vi "Take Measurement.vi"(6 "Angle of Attack":dbl, 8 "Setup filename":string="Wing_Pressure.xls", 9 "Averaging time (min)":dbl, 10 "File":T1, 11 "Filename":path) -> (0 "Array":cluster{dbl[], dbl[]}[](array[cluster]), 1 "Uref":dbl format="%#.3f", 2 "U Trav":dbl, 3 "Z":dbl)   [LabVIEW 2022 SP3]
uses:
  Anemometry/Anemometry Sub Vis/Controls/Save_Data.ctl
  Camera Server/Camera enum/Camera resolution.ctl
  Anemometry/Anemometry Sub Vis/Controls/Setup.ctl
  Anemometry/Anemometry Sub Vis/Globals/Meas_global.vi
  <vilib>/gmath/NI_Gmath.lvlib
panel:
  out "Lift/Drag":dbl format="%#.3f"
  out "CD":dbl format="%.3f"
  out "CL":dbl format="%.3f"
  out "Drag (N)":dbl format="%.3f"
  out "Lift (N)":dbl format="%.3f"
  out "Density Kg/m^3":dbl format="%#.3f"
  out "Fx Lower":dbl format="%#.3f"
  out "Fx Upper":dbl format="%#.3f"
  out "Fy Lower":dbl format="%#.2f"
  out "Fy Upper":dbl format="%#.2f"
  out "Fx (N)":dbl format="%.3f"
  out "Fy (N)":dbl format="%.3f"
  out "Fx":cluster{"xi used":dbl[], dbl[]}[](graph)
  out "Fy":cluster{"xi used":dbl[], dbl[]}[](graph)
  out "Pressure":cluster{dbl[], dbl[]}[](graph)
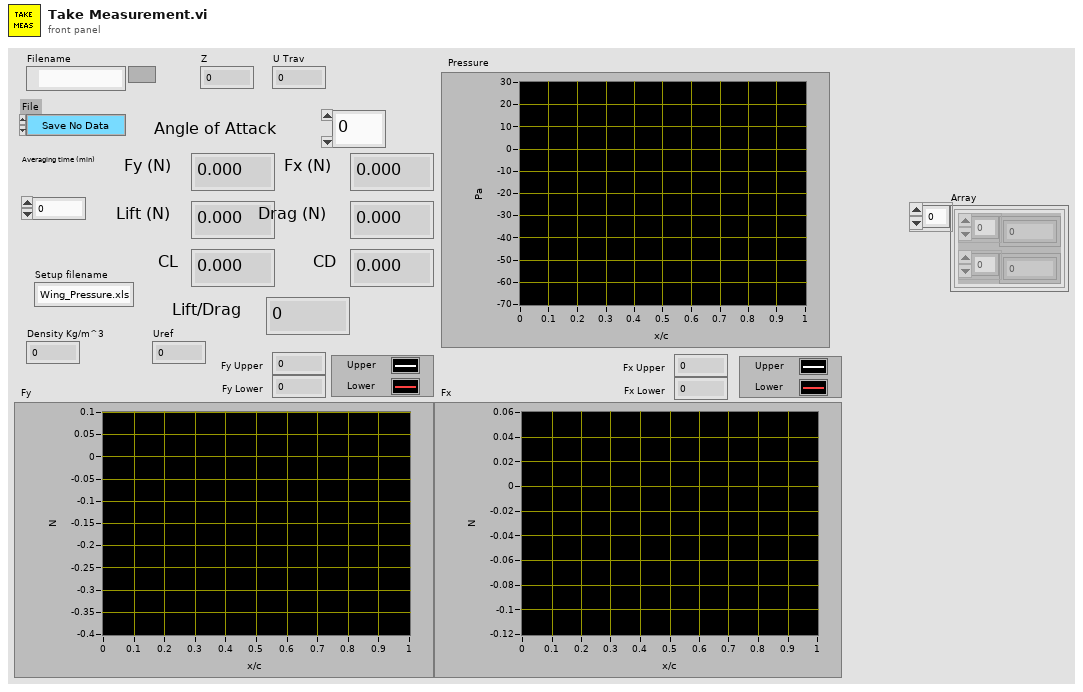
[diagram p1: front panel]
types:
  T1 = typedef "Save_Data.ctl" = enum16{"Save No Data", "Save Data"}
  T2 = typedef "Setup.ctl" = enum16{"Run Program", "Show Setup", "Save Current Setup", "Setup Front Panel"}
  T3 = typedef "Camera resolution.ctl" = u8
  T4 = typedef "Analysis_info_cluster.ctl" = cluster{"Colour":u32, "Inst type":T5, "Inst name":string, "Symbol":string, "Code name":string, "Extra Info":string, "Inst Array":T6, "Extra Titles":string[], "Extra Values":string[], "U":dbl, "u^2":dbl, "u^3":dbl, "u^4":dbl, "Skew_u":dbl, "Kurt_u":dbl, "Sd Error in Mean":dbl, "% u'/U":dbl, "X":dbl, "Y":dbl, "Z":dbl, "Timescale integral Estimate":dbl, "Sd Error in Variance":dbl, "Calib File":path, "Calib Constants":dbl[], "Output Position":bool, "Stats":enum16{"None", "Basic", "Full"}, "Av Sampling Rate":dbl, "Av No of Samples":dbl, "Total Meas Time (s)":dbl, "ADAM Ch Name":string, "Max value":dbl, "Min value":dbl, "Req Sample Rate Hz":dbl, "Sync Delay Time (s)":dbl, "Ch No":i16, "Device":string, "Use Latest Calib":bool, "Port":string, "Metadata Ch Names":string[], "Metadata Ch Values":string[], "Label":string}
  T5 = typedef "Inst_type.ctl" = enum16{"Raw voltage", "Raw with zero offsetting", "Propeller anemometer", "Pressure Transducer", "Pitot-static tube", "Hot wire", "Cross wire 1", "Cross wire 2", "Generic Linear", "Generic Polynomial", "Generic BackPoly", "Fast FID", "Thermocouple", "Cold wire", "Pulsed Wire", "LDA Vel", "LDA Tran time", "LDA Arr time", "Microphone"}
  T6 = typedef "Instrument_Array.ctl" = enum16{"PWA", "LDA", "Analogue"}
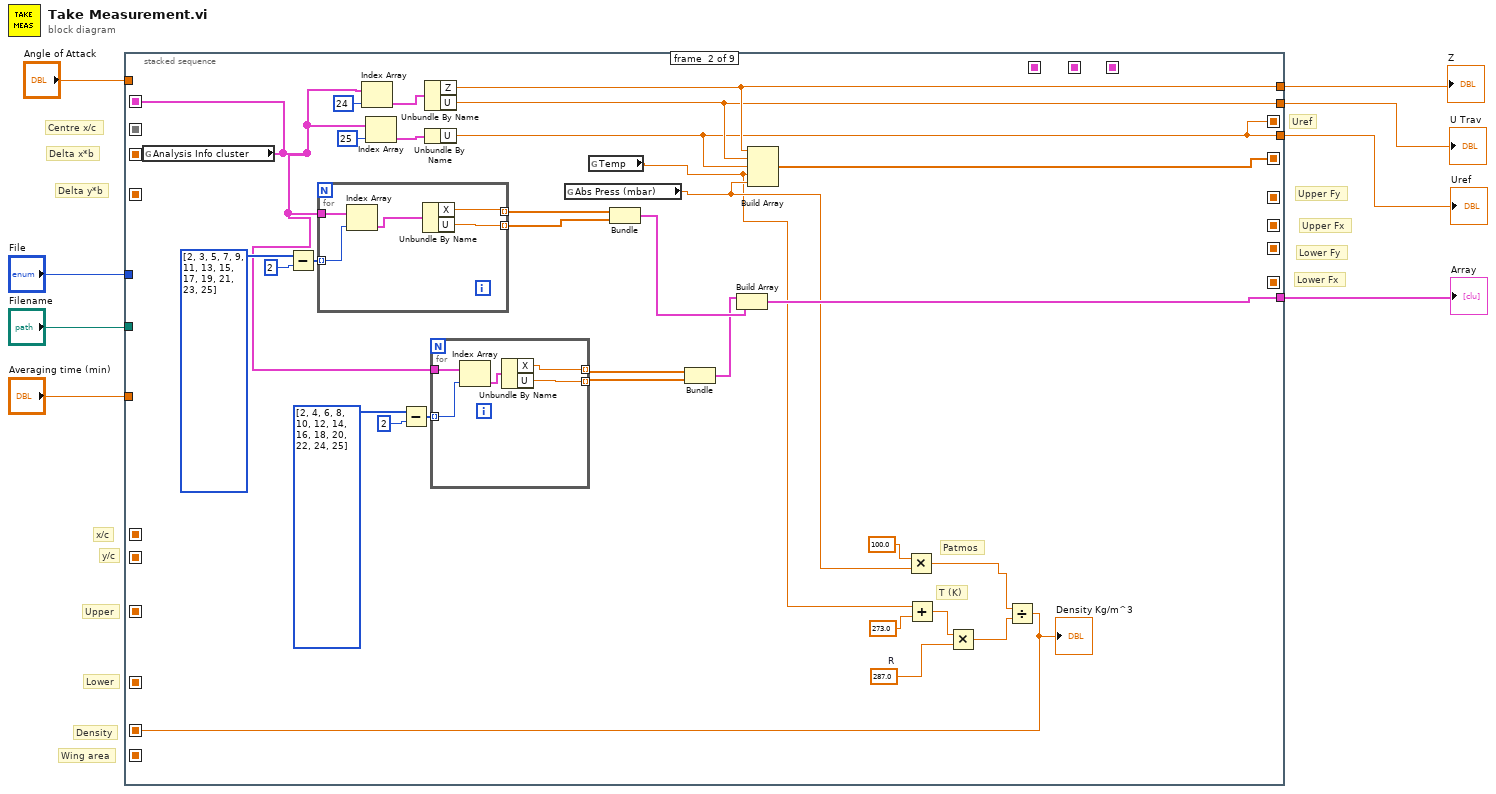
[diagram p0: block diagram]
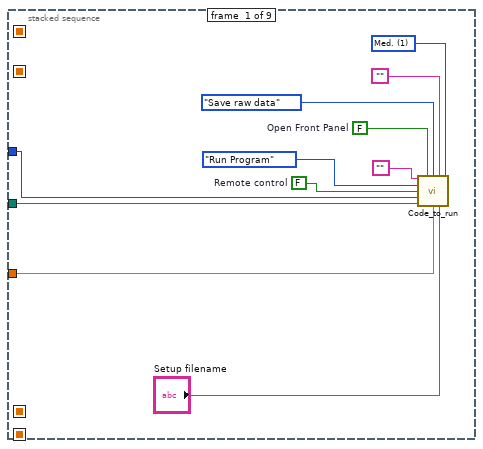
[diagram p2: hidden frame]
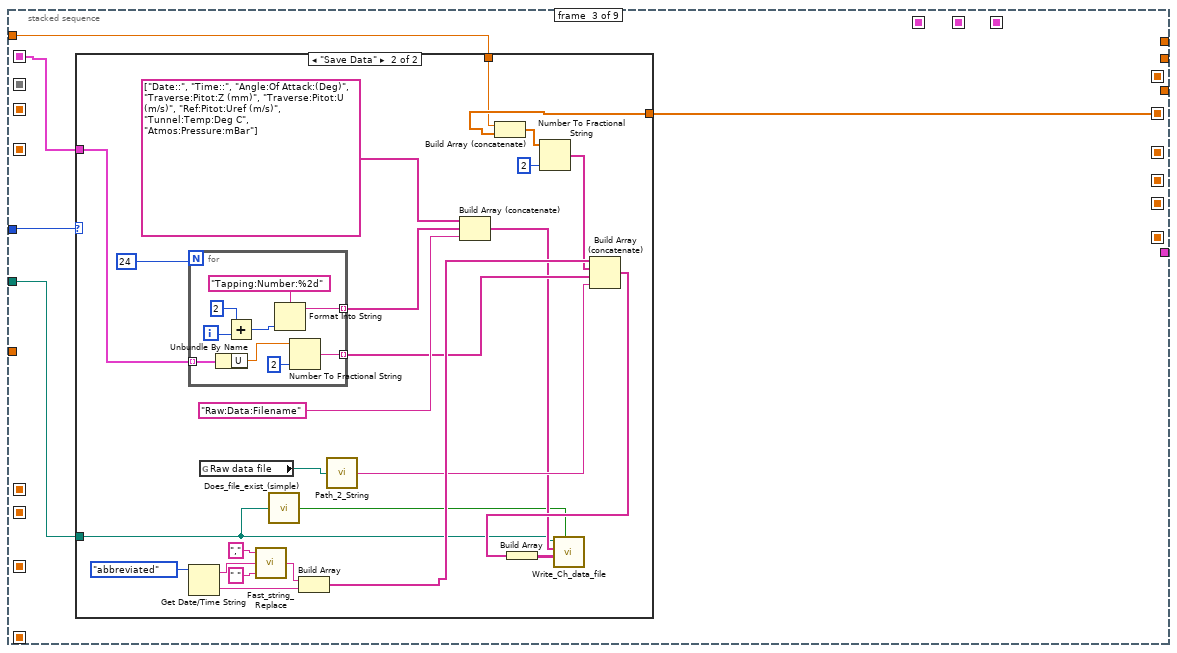
[diagram p3: hidden frame]
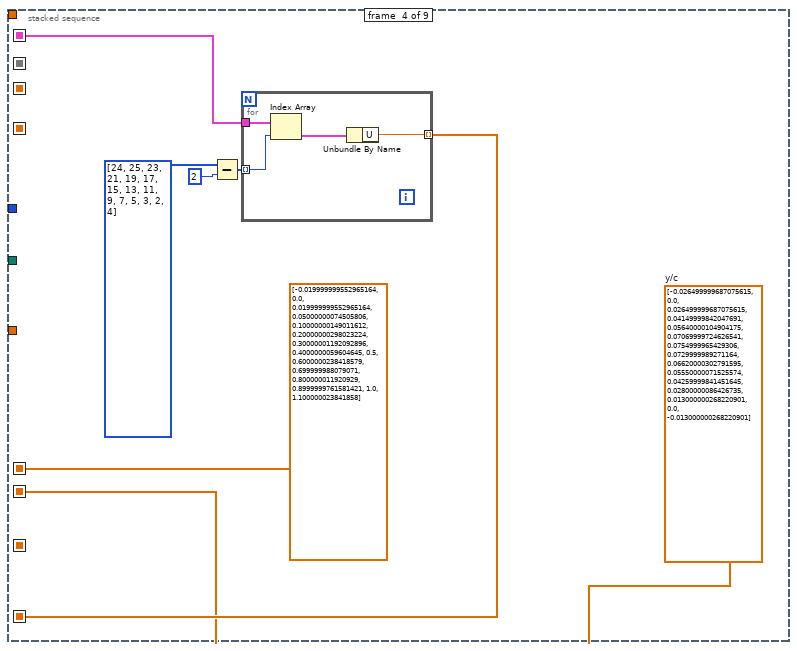
[diagram p5: hidden frame]
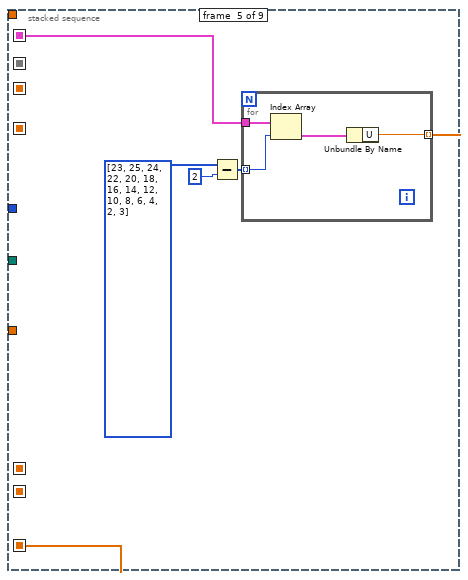
[diagram p6: hidden frame]
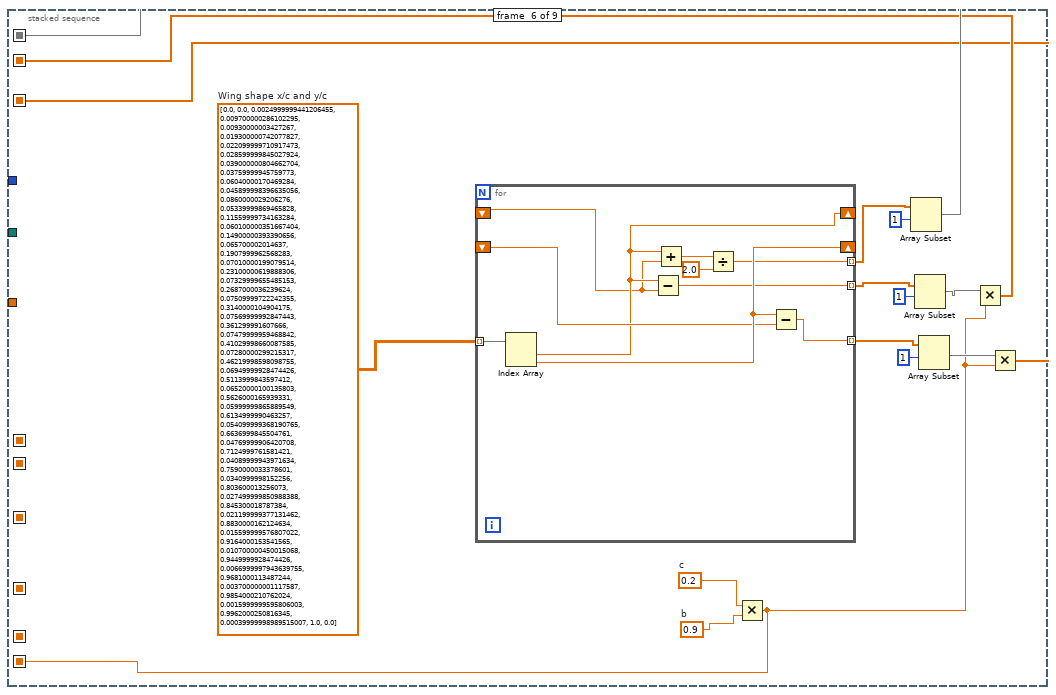
[diagram p7: hidden frame]
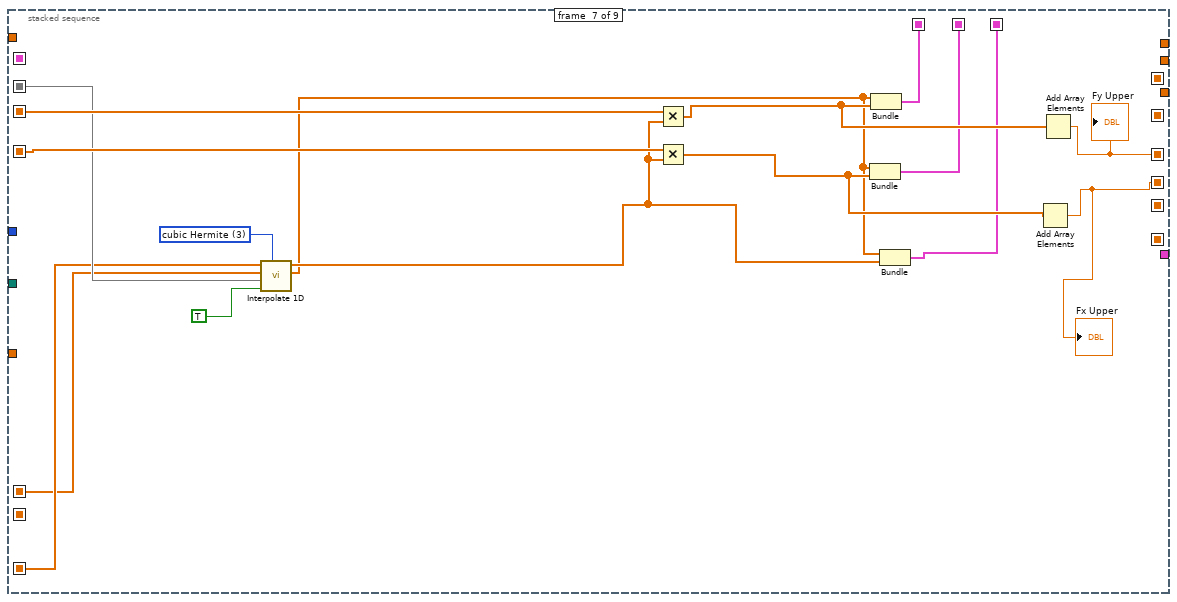
[diagram p8: hidden frame]
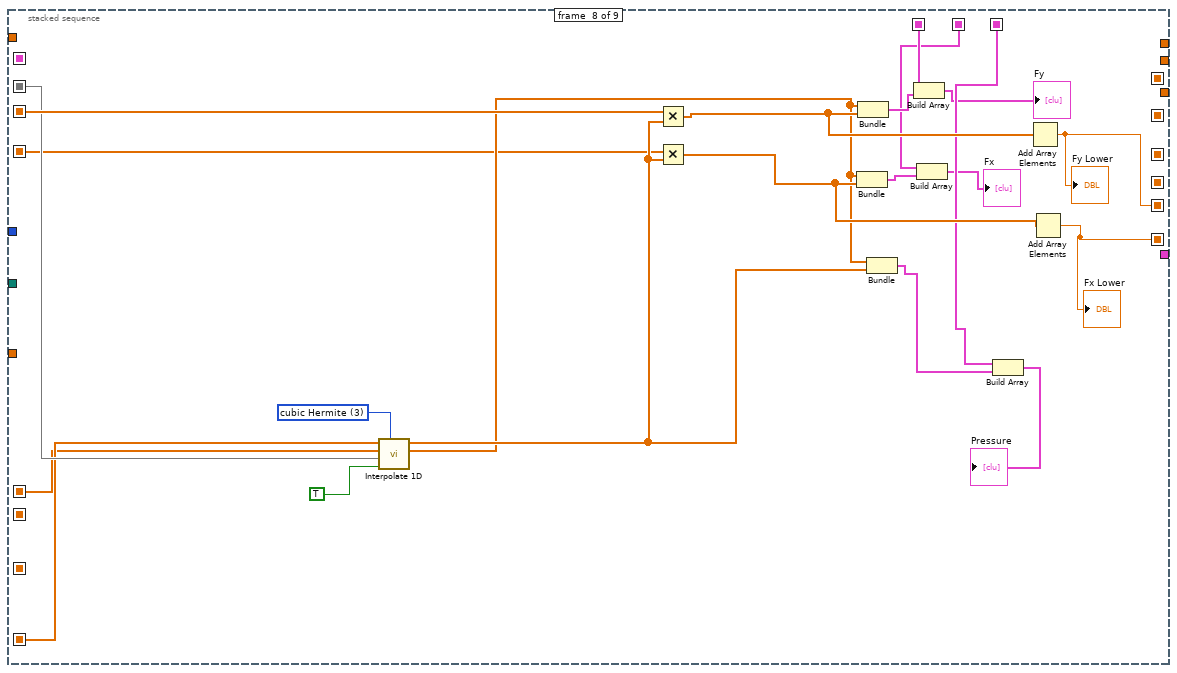
[diagram p9: hidden frame]
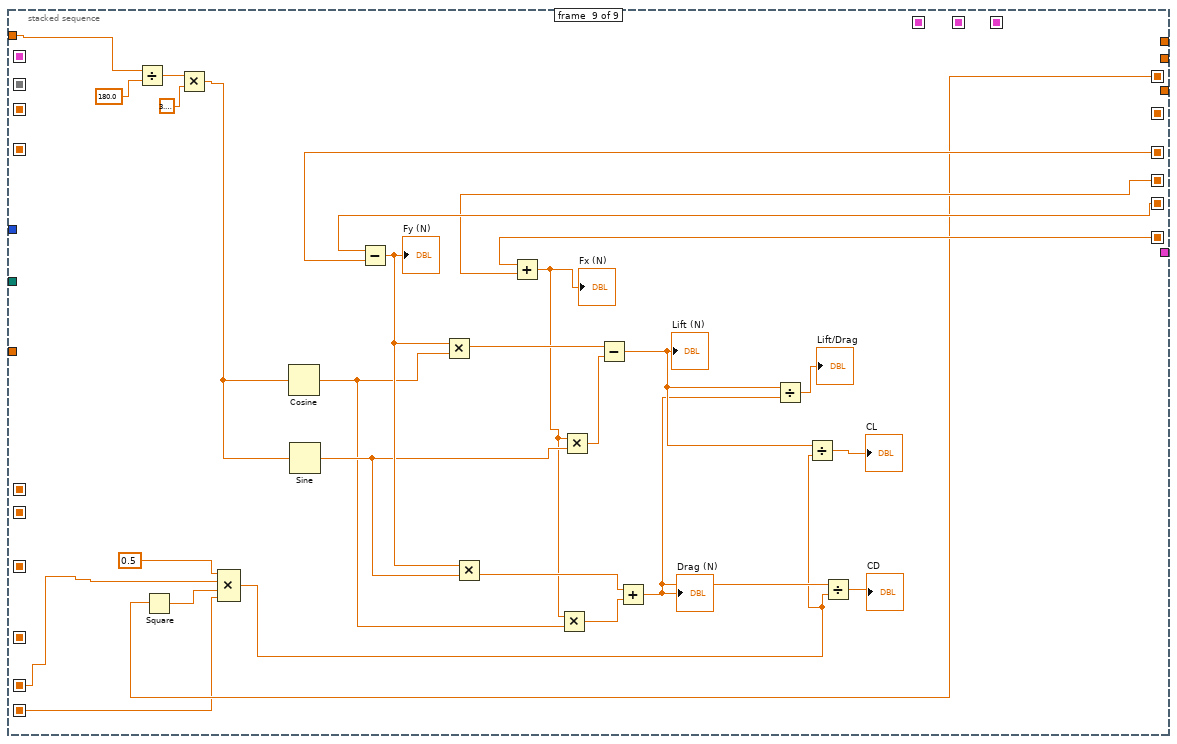
[diagram p10: hidden frame]
diagram:
  # "Wing area"
  # "Uref"
  # "Density"
  # "Lower Fx"
  # "Lower Fy"
  # "Upper Fx"
  # "Upper Fy"
  # "Delta y*b"
  # "Delta x*b"
  # "Centre x/c"
  # "y/c"
  # "x/c"
  # "Upper"
  # "Lower"
  n1 = stacked-sequence {
    seq-local: [_ w38 _ _ _ _ _ _ _] -> [_ _ w64 w103 w112 _ _ _ _]
    seq-local: [_ w32 _ _ _ _ _ _ _] -> [_ _ w63 _ _ _ _ _ _]
    seq-local: [_ _ _ w102 _ _ _ _ _] -> [_ _ _ _ _ _ _ w176 _]
    seq-local: [_ _ _ _ w111 _ _ _ _] -> [_ _ _ _ _ _ w152 _ _]
    seq-local: [_ _ _ dbl[] [-0.019999999552965164, 0.0, 0.019999999552965164, 0.05000000074505806, 0.10000000149011612, 0.20000000298023224, 0.30000001192092896, 0.4000000059604645, 0.5, 0.6000000238418579, 0.699999988079071, 0.800000011920929, 0.8999999761581421, 1.0, 1.100000023841858] _ _ _ _ _] -> [_ _ _ _ _ _ w151 w175 _]
    seq-local: [_ _ _ w100 _ _ _ _ _] -> [_ _ _ _ _ _ _ _ _]
    seq-local: [_ _ _ _ _ w131 _ _ _] -> [_ _ _ _ _ _ w158 w181 _]
    seq-local: [_ _ _ _ _ w123 _ _ _] -> [_ _ _ _ _ _ w160 w182 _]
    seq-local: [_ _ _ _ _ w121 _ _ _] -> [_ _ _ _ _ _ w159 w161 _]
    seq-local: [_ _ _ _ _ _ w156 _ _] -> [_ _ _ _ _ _ _ _ w209]
    seq-local: [_ _ _ _ _ _ w145 _ _] -> [_ _ _ _ _ _ _ _ w208]
    seq-local: [_ _ _ _ _ _ _ w163 _] -> [_ _ _ _ _ _ _ _ w210]
    seq-local: [_ _ _ _ _ _ _ w162 _] -> [_ _ _ _ _ _ _ _ w207]
    seq-local: [_ _ _ _ _ _ w148 _ _] -> [_ _ _ _ _ _ _ w167 _]
    seq-local: [_ _ _ _ _ _ w147 _ _] -> [_ _ _ _ _ _ _ w165 _]
    seq-local: [_ _ _ _ _ _ w146 _ _] -> [_ _ _ _ _ _ _ w170 _]
    seq-local: [_ w23 _ _ _ _ _ _ _] -> [_ _ _ _ _ _ _ _ w186]
    seq-local: [_ w22 _ _ _ _ _ _ _] -> [_ _ _ _ _ _ _ _ w185]
    seq-local: [_ _ _ _ _ w120 _ _ _] -> [_ _ _ _ _ _ _ _ w183]
    tunnel: "Filename" -> [w12 _ w62 _ _ _ _ _ _]
    tunnel: [_ w41 _ _ _ _ _ _ _] -> w3
    tunnel: [_ w22 _ _ _ _ _ _ _] -> w4
    tunnel: [_ w33 _ _ _ _ _ _ _] -> w5
    tunnel: [_ w34 _ _ _ _ _ _ _] -> w6
    tunnel: "Averaging time (min)" -> [w11 _ _ _ _ _ _ _ _]
    tunnel: "File" -> [w10 _ w65 _ _ _ _ _ _]
    tunnel: "Angle of Attack" -> [_ _ w61 _ _ _ _ _ w206]
    frame #0 {
      w17 = FALSE  # Remote control
      w14 = FALSE  # Open Front Panel
      w19 = T3 1 items=["Low", "Med.", "High", "Max."] ("Camera Resolution")
      n2 = call "Code_to_run.vi"("Extra command String"="", "Open Front Panel"=w14, "Raw data option"=enum16{"Save raw data", "Raw data not saved"}."Save raw data", "Current Row Comments"="", "Camera Resolution"=w19, "setup"=Setup."Run Program", "Remote control"=w17, "File"=w10, "Results Filename"=w12, "Averaging time (min)"=w11, "Setup filename"="Setup filename") -> ()  [unwired: 4 in, 1 out]
    }
    frame #1 {
      w26 = 287.0  # R
      # "T (K)"
      # "Patmos"
      n3 = global read "Meas_global.vi" "Analysis Info cluster"() -> (w38:T4[])
      n4 = Subtract(x=i32[] [2, 3, 5, 7, 9, 11, 13, 15, 17, 19, 21, 23, 25], y=2) -> (x-y=w49:i32[])
      n5 = for {
        tunnel: w38 -> [w60]
        tunnel: w49 -> [w59] mode=indexing
        tunnel: [w57] -> w37 mode=indexing
        tunnel: [w56] -> w46 mode=indexing
        n6 = Index Array(array=w60, index=w59) -> (element=w58:T4)
        n7 = Unbundle By Name(w58) -> ("X"=w56:dbl, "U"=w57:dbl)
      }
      n8 = Index Array(array=w38, index=24) -> (element=w42:T4)
      n9 = Index Array(array=w38, index=25) -> (element=w44:T4)
      n10 = Subtract(x=i32[] [2, 4, 6, 8, 10, 12, 14, 16, 18, 20, 22, 24, 25], y=2) -> (x-y=w48:i32[])
      n11 = Unbundle By Name(w42) -> ("Z"=w34:dbl, "U"=w33:dbl)
      n12 = Unbundle By Name(w44) -> ("U"=w22:dbl)
      n13 = for {
        tunnel: w38 -> [w55]
        tunnel: w48 -> [w54] mode=indexing
        tunnel: [w52] -> w35 mode=indexing
        tunnel: [w51] -> w36 mode=indexing
        n14 = Index Array(array=w55, index=w54) -> (element=w53:T4)
        n15 = Unbundle By Name(w53) -> ("X"=w51:dbl, "U"=w52:dbl)
      }
      n16 = global read "Meas_global.vi" "Abs Press (mbar)"() -> (w31:dbl)
      n17 = global read "Meas_global.vi" "Temp"() -> (w29:dbl)
      n18 = Bundle(w46, w37) -> (w21:cluster{dbl[], dbl[]})  [unwired: 1 in]
      n19 = Bundle(w36, w35) -> (w20:cluster{dbl[], dbl[]})  [unwired: 1 in]
      n20 = Build Array(w20, w21) -> (w41:cluster{dbl[], dbl[]}[])
      n21 = Build Array(w34, w33, w22, w29, w31) -> (w32:dbl[])
      n22 = Multiply(x=100.0, y=w31) -> (x*y=w24:dbl)
      n23 = Add(x=w29, y=273.0) -> (x+y=w27:dbl)
      n24 = Multiply(x=w27, y=w26) -> (x*y=w25:dbl)
      n25 = Divide(x=w24, y=w25) -> (x/y=w23:dbl)
      "Density Kg/m^3" <- w23
    }
    frame #2 {
      n26 = case shown="\"Save Data\"" w65 {
        tunnel: w64 -> [_ w77]
        tunnel: w63 -> [_ w70]
        tunnel: w62 -> [_ w68]
        tunnel: w61 -> [_ w66]
        frame "Save No Data", Default {
        }
        frame "Save Data" {
          n27 = for {
            N: 24 -> [_]
            tunnel: [w95] -> w88 mode=indexing
            tunnel: w77 -> [w94] mode=indexing
            tunnel: [w91] -> w76 mode=indexing
            i -> [w99]
            n28 = Unbundle By Name(w94) -> ("U"=w92:dbl)
            n29 = Add(x=2, y=w99) -> (x+y=w97:i32)
            n30 = Format Into String(format string="Tapping:Number:%2d", w97) -> (resulting string=w95:string)  [unwired: 2 in, 1 out]
            n31 = Number To Fractional String(number=w92, precision (6)=i16 2) -> (F-format string=w91:string)  [unwired: 2 in]
          }
          n32 = Get Date/Time String(date format (0)=enum16{"short", "long", "abbreviated"}."abbreviated") -> (date string=w86:string, time string=w81:string)  [unwired: 2 out]
          n33 = global read "Meas_global.vi" "Raw data file"() -> (w75:path)
          n34 = call "Fast_string_Replace.vi"("Replace match with:"=" ", "Input String"=w86, "matchThis"="," ("regular expression")) -> ("Output String"=w82:string)  [unwired: 1 in, 1 out]
          n35 = call "Does_file_exist_(simple).vi"("Pathname"=w68) -> ("exists?"=w67:bool)
          n36 = Build Array(w82, w81) -> (w79:string[])
          n37 = call "Path_2_String.vi"("Real Path"=w75) -> ("Path String"=w74:string)
          n38 = Build Array (concatenate)(string[] ["Date::", "Time::", "Angle:Of Attack:(Deg)", "Traverse:Pitot:Z (mm)", "Traverse:Pitot:U (m/s)", "Ref:Pitot:Uref (m/s)", "Tunnel:Temp:Deg C", "Atmos:Pressure:mBar"], w88, "Raw:Data:Filename") -> (w71:string[])
          n39 = Build Array (concatenate)(w66, w70) -> (w69:dbl[])
          n40 = Number To Fractional String(number=w69, precision (6)=i16 2) -> (F-format string=w78:string[])  [unwired: 2 in]
          n41 = Build Array (concatenate)(w79, w78, w76, w74) -> (w73:string[])
          n42 = Build Array(w73) -> (w72:string[][])
          n43 = call "Write_Ch_data_file.vi"("exists?"=w67, "Channel Values"=w72, "Channel names"=w71, "Filename"=w68) -> ()  [unwired: 4 in, 4 out]
        }
      }
    }
    frame #3 {
      w100 = dbl[] [-0.026499999687075615, 0.0, 0.026499999687075615, 0.04149999842047691, 0.05640000104904175, 0.07069999724626541, 0.0754999965429306, 0.0729999989271164, 0.06620000302791595, 0.05550000071525574, 0.04259999841451645, 0.02800000086426735, 0.013000000268220901, 0.0, -0.013000000268220901]  # y/c
      n44 = Subtract(x=i32[] [24, 25, 23, 21, 19, 17, 15, 13, 11, 9, 7, 5, 3, 2, 4], y=2) -> (x-y=w105:i32[])
      n45 = for {
        tunnel: w103 -> [w110]
        tunnel: w105 -> [w109] mode=indexing
        tunnel: [w107] -> w102 mode=indexing
        n46 = Index Array(array=w110, index=w109) -> (element=w108:T4)
        n47 = Unbundle By Name(w108) -> ("U"=w107:dbl)
      }
    }
    frame #4 {
      n48 = Subtract(x=i32[] [23, 25, 24, 22, 20, 18, 16, 14, 12, 10, 8, 6, 4, 2, 3], y=2) -> (x-y=w114:i32[])
      n49 = for {
        tunnel: w112 -> [w119]
        tunnel: w114 -> [w118] mode=indexing
        tunnel: [w116] -> w111 mode=indexing
        n50 = Index Array(array=w119, index=w118) -> (element=w117:T4)
        n51 = Unbundle By Name(w117) -> ("U"=w116:dbl)
      }
    }
    frame #5 {
      w125 = 0.9  # b
      w126 = 0.2  # c
      w134 = sgl[][] [[0.0, 0.0], [0.0025, 0.0097], [0.0093, 0.0193], [0.0221, 0.0286], [0.039, 0.0376], [0.0604, 0.0459], [0.086, 0.0534], [0.1156, 0.0601], [0.149, 0.0657], [0.1908, 0.0701], [0.231, 0.0733], [0.2687, 0.0751], [0.314, 0.0757], [0.3613, 0.0748], [0.4103, 0.0728], [0.4622, 0.0695], [0.5114, 0.0652], [0.5626, 0.06], [0.6135, 0.0541], [0.6637, 0.0477], [0.7125, 0.0409], [0.759, 0.0341], [0.8036, 0.0275], [0.8453, 0.0212], [0.883, 0.0156], [0.9164, 0.0107], [0.945, 0.0067], [0.9681, 0.0037], [0.9854, 0.0016], [0.9962, 0.0004], [1.0, 0.0]]  # Wing shape x/c and y/c
      n52 = for {
        tunnel: w134 -> [w144] mode=indexing
        shift-right: [w141] -> _
        shift-left: _ -> [w140]
        shift-right: [w143] -> _
        shift-left: _ -> [w142]
        tunnel: [w137] -> w132 mode=indexing
        tunnel: [w136] -> w129 mode=indexing
        tunnel: [w135] -> w128 mode=indexing
        n53 = Index Array(array=w144) -> (element #1=w141:sgl, element #2=w143:sgl)  [unwired: 2 in]
        n54 = Subtract(x=w141, y=w140) -> (x-y=w136:sgl)
        n55 = Add(x=w141, y=w140) -> (x+y=w139:sgl)
        n56 = Divide(x=w139, y=sgl 2.0) -> (x/y=w137:sgl)
        n57 = Subtract(x=w143, y=w142) -> (x-y=w135:sgl)
      }
      n58 = Multiply(x=w126, y=w125) -> (x*y=w120:dbl)
      n59 = Array Subset(array=w132, index=1) -> (w131:sgl[])  [unwired: 1 in]
      n60 = Array Subset(array=w129, index=1) -> (w124:sgl[])  [unwired: 1 in]
      n61 = Array Subset(array=w128, index=1) -> (w122:sgl[])  [unwired: 1 in]
      n62 = Multiply(x=w124, y=w120) -> (x*y=w123:dbl[])
      n63 = Multiply(x=w122, y=w120) -> (x*y=w121:dbl[])
    }
    frame #6 {
      w154 = 3 items=["nearest", "linear", "spline", "cubic Hermite", "Lagrange"] ("method")
      n64 = call <vilib>:"Interpolate 1D.vi"("method"=w154, "X is monotonic"=TRUE, "xi"=w158, "X"=w151, "Y"=w152) -> ("xi used"=w149:dbl[], "yi"=w150:dbl[])  [unwired: 4 in, 1 out]
      n65 = Multiply(x=w160, y=w150) -> (x*y=w157:dbl[])
      n66 = Multiply(x=w159, y=w150) -> (x*y=w155:dbl[])
      n67 = Bundle("xi used"=w149, w155) -> (w147:cluster{"xi used":dbl[], dbl[]})  [unwired: 1 in]
      n68 = Bundle("xi used"=w149, w157) -> (w148:cluster{"xi used":dbl[], dbl[]})  [unwired: 1 in]
      n69 = Bundle("xi used"=w149, "yi"=w150) -> (w146:cluster{"xi used":dbl[], "yi":dbl[]})  [unwired: 1 in]
      n70 = Add Array Elements(numeric array=w155) -> (sum=w145:dbl)
      "Fx Upper" <- w145
      n71 = Add Array Elements(numeric array=w157) -> (sum=w156:dbl)
      "Fy Upper" <- w156
    }
    frame #7 {
      w172 = 3 items=["nearest", "linear", "spline", "cubic Hermite", "Lagrange"] ("method")
      n72 = call <vilib>:"Interpolate 1D.vi"("method"=w172, "X is monotonic"=TRUE, "xi"=w181, "X"=w175, "Y"=w176) -> ("xi used"=w173:dbl[], "yi"=w174:dbl[])  [unwired: 4 in, 1 out]
      n73 = Multiply(x=w182, y=w174) -> (x*y=w178:dbl[])
      n74 = Multiply(x=w161, y=w174) -> (x*y=w177:dbl[])
      n75 = Bundle("xi used"=w173, w177) -> (w169:cluster{"xi used":dbl[], dbl[]})  [unwired: 1 in]
      n76 = Bundle("xi used"=w173, w178) -> (w168:cluster{"xi used":dbl[], dbl[]})  [unwired: 1 in]
      n77 = Bundle("xi used"=w173, "yi"=w174) -> (w180:cluster{"xi used":dbl[], "yi":dbl[]})  [unwired: 1 in]
      n78 = Build Array(w167, w168) -> (→"Fy":cluster{"xi used":dbl[], dbl[]}[])
      n79 = Build Array(w165, w169) -> (→"Fx":cluster{"xi used":dbl[], dbl[]}[])
      n80 = Build Array(w170, w180) -> (→"Pressure":cluster{"xi used":dbl[], "yi":dbl[]}[])
      n81 = Add Array Elements(numeric array=w178) -> (sum=w163:dbl)
      "Fy Lower" <- w163
      n82 = Add Array Elements(numeric array=w177) -> (sum=w162:dbl)
      "Fx Lower" <- w162
    }
    frame #8 {
      n83 = Divide(x=w206, y=180.0) -> (x/y=w204:dbl)
      n84 = Square(x=w185) -> (x^2=w188:dbl)
      n85 = Multiply(x=w204, y=3.141592653589793) -> (x*y=w202:dbl)
      n86 = Compound Arithmetic op=MULTIPLY(0.5, w186, w188, w183) -> (w184:dbl)
      n87 = Cosine(x=w202) -> (cos(x)=w195:dbl)
      n88 = Sine(x=w202) -> (sin(x)=w198:dbl)
      n89 = Subtract(x=w210, y=w209) -> (x-y=w199:dbl)
      "Fy (N)" <- w199
      n90 = Multiply(x=w199, y=w195) -> (x*y=w201:dbl)
      n91 = Multiply(x=w199, y=w198) -> (x*y=w197:dbl)
      n92 = Add(x=w207, y=w208) -> (x+y=w196:dbl)
      "Fx (N)" <- w196
      n93 = Multiply(x=w196, y=w195) -> (x*y=w194:dbl)
      n94 = Multiply(x=w196, y=w198) -> (x*y=w200:dbl)
      n95 = Subtract(x=w201, y=w200) -> (x-y=w191:dbl)
      "Lift (N)" <- w191
      n96 = Add(x=w197, y=w194) -> (x+y=w190:dbl)
      "Drag (N)" <- w190
      n97 = Divide(x=w191, y=w190) -> (x/y=→"Lift/Drag":dbl)
      n98 = Divide(x=w191, y=w184) -> (x/y=→"CL":dbl)
      n99 = Divide(x=w190, y=w184) -> (x/y=→"CD":dbl)
    }
  }
  "Z" <- w6
  "U Trav" <- w5
  "Uref" <- w4
  "Array" <- w3
